vi "Write nextInChain.vi"(8 "error in (no error)":errorcluster, 10 "Chain.lvclass":refnum<class "Chain.lvclass">, 11 "Multiply in":refnum<class "Multiply.lvclass">) -> (0 "error out":errorcluster, 3 "Multiply out":refnum<class "Multiply.lvclass">)   [LabVIEW 2017, in "Multiply.lvclass"]
uses:
  Multiply.lvclass
  Chain Class/Chain.lvclass
  Multiply.lvclass/Multiply.ctl
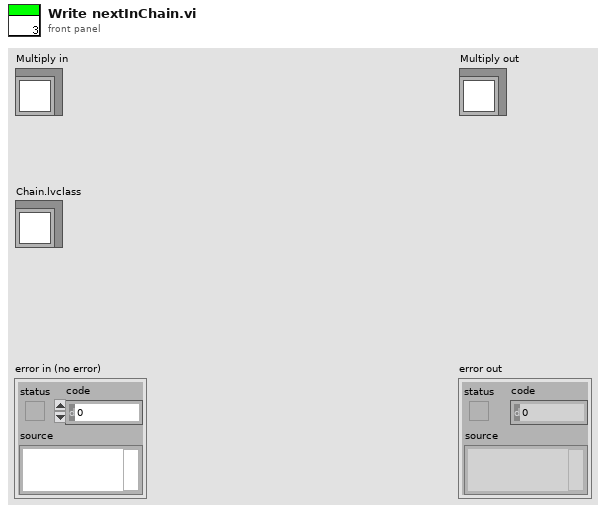
[diagram p1: front panel]
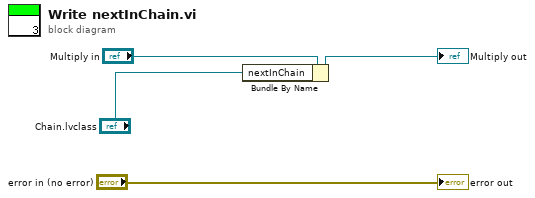
[diagram p0: block diagram]
diagram:
  n1 = Bundle By Name(cluster="Multiply in", "nextInChain"="Chain.lvclass") -> (→"Multiply out":refnum<class "Multiply.lvclass">)
  "error out" <- "error in (no error)"
